vi "pre_filter_image_8bit_dll.vi"(7 "Gaussian Filter Size":dbl, 8 "error in (no error)":errorcluster, 9 "Mean Filter Size":i32, 11 "Input Image":T1) -> (0 "error out":errorcluster, 2 "Output Image Array":dbl[][](array[numeric]))   [LabVIEW 2016]
doc: "Calls DLL to apply pre-filtering to image prior to speckle correlalation measurements. Image is filtered using 'pre-filter' in raptor.dll. A mean filtered copy of the image is subtracted and then a Gaussian Filter is applied."
uses:
  <vilib>/vision/Image Controls.llb/IMAQ Image.ctl
  Raptor.dll
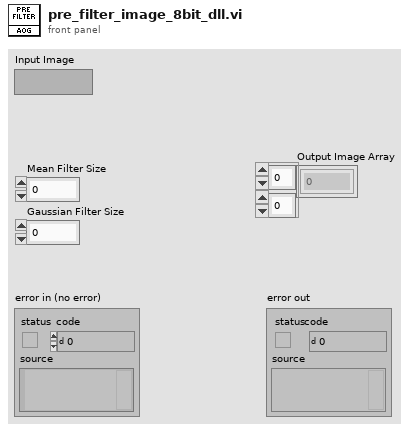
[diagram p1: front panel]
types:
  T1 = typedef "IMAQ Image.ctl" = refnum<image>
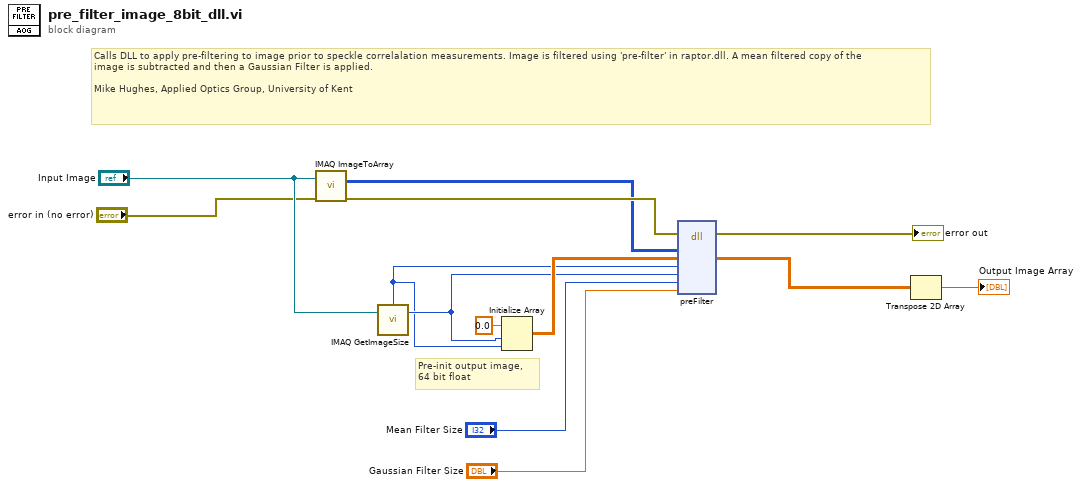
[diagram p0: block diagram]
diagram:
  # "Pre-init output image, \n64 bit float"
  # "Calls DLL to apply pre-filtering to image prior to speckle correlalation measurements. Image is filtered using 'pre-filter' in raptor.dll. A mean filtered copy of the\nimage is subtracted and then a Gaussian Filter is applied.\n\nMike Hughes, Applied Optics Group, University of Kent"
  n1 = call "IMAQ ImageToArray"("error in (no error)"="error in (no error)", "Image"="Input Image") -> ("error out"=w8:errorcluster, "Image Pixels (U8)"=w6:u8[][])  [unwired: 2 in, 3 out]
  n2 = call "IMAQ GetImageSize"("Image"="Input Image") -> ("Y Resolution"=w5:i32, "X Resolution"=w4:i32)  [unwired: 3 in, 1 out]
  n3 = Initialize Array(0.0 ("element"), w5, w4) -> (w11:dbl[][])
  n4 = dll-call lib="\\\\healey\\aog/general storage/REBOT/code/volume_assembly/Labview Raptor/Raptor3/lib/Raptor.dll" fn="preFilter"(error in=w8, "im_in"=w6, "im_out"=w11, "img_cols"=w4, "img_rows"=w5, "meanFilterSize"="Mean Filter Size", "gaussFilterSize"="Gaussian Filter Size") -> (error out=→"error out":errorcluster, "im_out"=w2:dbl[][])  [unwired: 8 in, 1 out]
  n5 = Transpose 2D Array(2D array=w2) -> (transposed array=→"Output Image Array":dbl[][])
